vi "Autonomous Independent.vi"   [LabVIEW 2018]
doc: "This VI is called when autonomous begins, and will automatically be terminated when autonomous ends. You can carry out timed or sensor driven robot movement independently without needing to return to the caller."
uses:
  <vilib>/Rock Robotics/WPI/Utilities/WPI_GetSetVariantRefNum.vi
  <vilib>/Rock Robotics/Network Tables/NT Read String.vi
  <vilib>/Rock Robotics/Network Tables/NT Write Numeric Array.vi
panel:
  # "Be sure to right-click and choose Data Operations>>Make Current Value default if you want to save the array values with the VI"
types:
  T1 = typedef "WPI_JoystickDevRef.ctl" = cluster{"Device":T2}
  T2 = typedef "WPI_JoystickDeviceEnum.ctl" = enum16{"USB 0", "USB 1", "USB 2", "USB 3", "USB 4", "USB 5"}
  T3 = cluster{"Gyro":string, "Mtr 1":string, "Mtr 2":string}
  T4 = typedef "WPI_RobotDriveDevRef.ctl" = cluster{"DevStatus":errorcluster, "Motors[]":T5[], "Square Inputs":bool, "Max Output":dbl}
  T5 = typedef "WPI_MotorControlDeviceRef.ctl" = cluster{"DeviceStatus":errorcluster, "Type":T6, "PWM":cluster{"PWM Channel":T7, "DeadBand":T8}, "CAN":cluster{"Device Number":u8, "SetOutput VI Ref":variant, "GetOutput VI Ref":variant, "Enable VI Ref":variant, "Disable VI Ref":variant, "Data":variant}, "Invert":bool, "DIO PWM":cluster{"PWM \"Enable\" Channel":T7, "DIOChannel":T9, "PWM Rate":dbl}}
  T6 = typedef "WPI_MotorControlType.ctl" = enum16{"PWM", "CAN", "DIO PWM"}
  T7 = typedef "FPGA_DIOPWMChannel.ctl" = enum8{"PWM 0", "PWM 1", "PWM 2", "PWM 3", "PWM 4", "PWM 5", "PWM 6", "PWM 7", "PWM 8", "PWM 9", "PWM MXP 0", "PWM MXP 1", "PWM MXP 2", "PWM MXP 3", "PWM MXP 4", "PWM MXP 5", "PWM MXP 6", "PWM MXP 7", "PWM MXP 8", "PWM MXP 9", "Invalid"}
  T8 = typedef "WPI_PWMDeadband.ctl" = cluster{"Name":string, "maxPositivePwm":i32, "minPositivePwm":i32, "centerPwm":i32, "maxNegativePwm":i32, "minNegativePwm":i32, "angularRange":u16}
  T9 = typedef "FPGA_DIOChannel.ctl" = enum8{"DIO 0", "DIO 1", "DIO 2", "DIO 3", "DIO 4", "DIO 5", "DIO 6", "DIO 7", "DIO 8", "DIO 9", "DIO MXP 0", "DIO MXP 1", "DIO MXP 2", "DIO MXP 3", "DIO MXP 4", "DIO MXP 5", "DIO MXP 6", "DIO MXP 7", "DIO MXP 8", "DIO MXP 9", "DIO MXP 10", "DIO MXP 11", "DIO MXP 12", "DIO MXP 13", "DIO MXP 14", "DIO MXP 15", "SPI Port CS1", "SPI Port CS2", "SPI Port CS3", "SPI Port MISO", "SPI Port MOSI", "Invalid"}
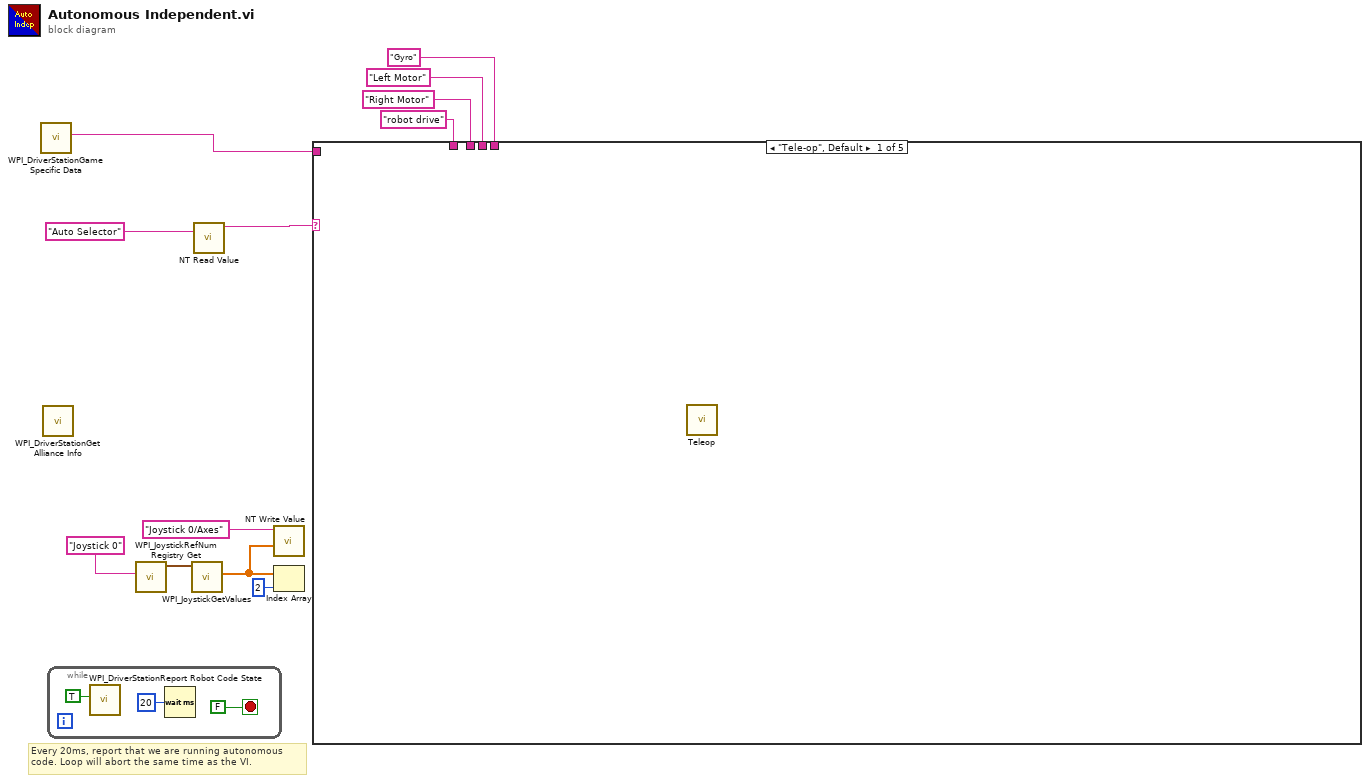
[diagram p0: block diagram]
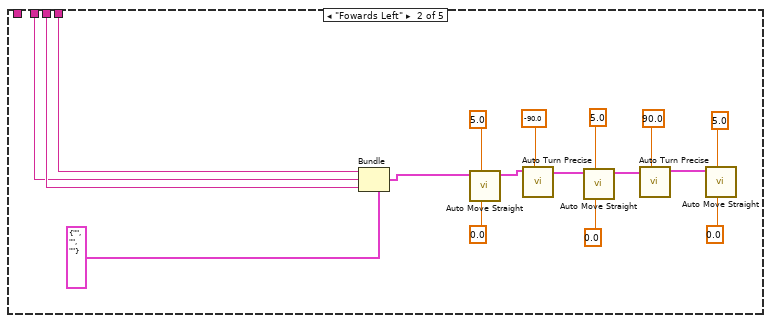
[diagram p2: hidden frame]
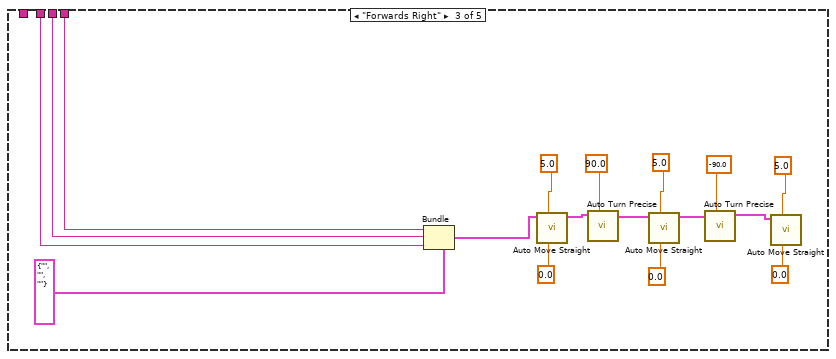
[diagram p3: hidden frame]
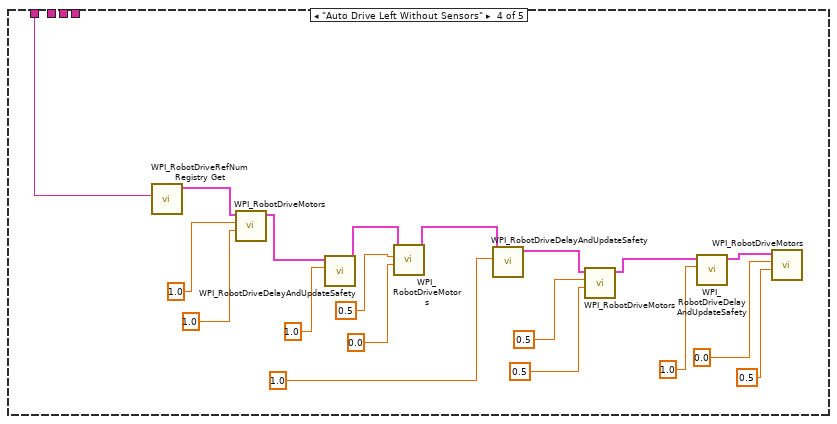
[diagram p4: hidden frame]
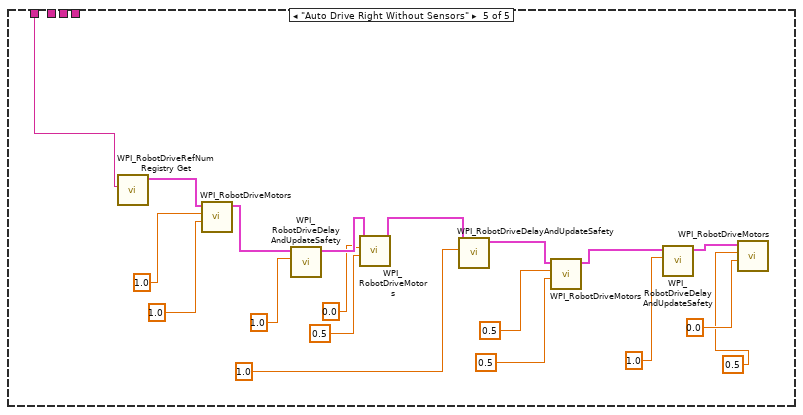
[diagram p5: hidden frame]
diagram:
  # "Every 20ms, report that we are running autonomous\ncode. Loop will abort the same time as the VI."
  n1 = call <vilib>:"WPI_DriverStationGame Specific Data.vi"() -> ("Game Specific Data"=w5:string)  [unwired: 11 in]
  n2 = call <vilib>:"WPI_DriverStationGet Alliance Info.vi"() -> ()  [unwired: 12 out]
  n3 = while {
    stop <- FALSE stop-if-true
    n4 = call <vilib>:"WPI_DriverStationReport Robot Code State.vi"("Autonomous"=TRUE) -> ()  [unwired: 10 in, 1 out]
    n5 = Wait (ms)(milliseconds to wait=u32 20) -> ()  [unwired: 1 out]
  }
  n6 = call <vilib>:"WPI_JoystickRefNum Registry Get.vi"("refnum name"="Joystick 0") -> ("JoystickDevRef"=w11:T1)  [unwired: 1 in, 9 out]
  n7 = call <vilib>:"WPI_JoystickGetValues.vi"("JoystickDevRef"=w11) -> ("Axes"=w7:dbl[])  [unwired: 6 in, 4 out]
  n8 = call-poly <vilib>:"NT Read Value.vi"("Name"="Auto Selector") -> ("String"=w8:string)  [unwired: 9 in, 1 out]
  n9 = call-poly <vilib>:"NT Write Value.vi"("Numeric Array"=w7, "Name"="Joystick 0/Axes") -> ()  [unwired: 9 in, 1 out]
  n10 = Index Array(array=w7, index=2) -> ()  [unwired: 1 out]
  n11 = case shown="\"Tele-op\", Default" w8 {
    tunnel: w5 -> [_ _ _ _ _]
    tunnel: "robot drive" ("refnum name") -> [_ _ _ w50 w69]
    tunnel: "Gyro" ("refnum name") -> [_ w18 w35 _ _]
    tunnel: "Left Motor" ("refnum name") -> [_ w17 w33 _ _]
    tunnel: "Right Motor" ("refnum name") -> [_ w16 w34 _ _]
    frame "Tele-op", Default {
      n12 = call "Teleop.vi"() -> ()  [unwired: 3 in, 9 out]
    }
    frame "Fowards Left" {
      n13 = Bundle(cluster=T3 {"Gyro"="", "Mtr 1"="", "Mtr 2"=""} ("Refnum's In"), "Gyro"=w18, "Mtr 1"=w16, "Mtr 2"=w17) -> (w21:T3)
      n14 = call "Auto Move Straight.vi"("Target Angle"=0.0, "Target Distance"=5.0, "Refnum's In"=w21) -> ("Refnum's Out"=w29:T3)  [unwired: 7 in, 1 out]
      n15 = call "Auto Turn Precise.vi"("Target Distance"=-90.0, "Refnum's In"=w29) -> ("Refnum's Out"=w28:T3)  [unwired: 8 in, 1 out]
      n16 = call "Auto Move Straight.vi"("Target Angle"=0.0, "Target Distance"=5.0, "Refnum's In"=w28) -> ("Refnum's Out"=w26:T3)  [unwired: 7 in, 1 out]
      n17 = call "Auto Turn Precise.vi"("Target Distance"=90.0, "Refnum's In"=w26) -> ("Refnum's Out"=w24:T3)  [unwired: 8 in, 1 out]
      n18 = call "Auto Move Straight.vi"("Target Angle"=0.0, "Target Distance"=5.0, "Refnum's In"=w24) -> ()  [unwired: 7 in, 2 out]
    }
    frame "Forwards Right" {
      n19 = Bundle(cluster=T3 {"Gyro"="", "Mtr 1"="", "Mtr 2"=""} ("Refnum's In"), "Gyro"=w35, "Mtr 1"=w34, "Mtr 2"=w33) -> (w45:T3)
      n20 = call "Auto Move Straight.vi"("Target Angle"=0.0, "Target Distance"=5.0, "Refnum's In"=w45) -> ("Refnum's Out"=w44:T3)  [unwired: 7 in, 1 out]
      n21 = call "Auto Turn Precise.vi"("Target Distance"=90.0, "Refnum's In"=w44) -> ("Refnum's Out"=w43:T3)  [unwired: 8 in, 1 out]
      n22 = call "Auto Move Straight.vi"("Target Angle"=0.0, "Target Distance"=5.0, "Refnum's In"=w43) -> ("Refnum's Out"=w40:T3)  [unwired: 7 in, 1 out]
      n23 = call "Auto Turn Precise.vi"("Target Distance"=-90.0, "Refnum's In"=w40) -> ("Refnum's Out"=w38:T3)  [unwired: 8 in, 1 out]
      n24 = call "Auto Move Straight.vi"("Target Angle"=0.0, "Target Distance"=5.0, "Refnum's In"=w38) -> ()  [unwired: 7 in, 2 out]
    }
    frame "Auto Drive Left Without Sensors" {
      n25 = call <vilib>:"WPI_RobotDriveRefNum Registry Get.vi"("refnum name"=w50) -> ("RobotDriveDevRef"=w61:T4)  [unwired: 9 in, 1 out]
      n26 = call <vilib>:"WPI_RobotDriveMotors.vi"("RightSpeed"=1.0 ("Y axis value"), "LeftSpeed"=1.0 ("X axis value"), "RobotDriveDevRef"=w61) -> ("RobotDriveDevRef"=w60:T4)  [unwired: 6 in, 2 out]
      n27 = call <vilib>:"WPI_RobotDriveDelayAndUpdateSafety.vi"("Delay (s)"=1.0, "RobotDriveDevRef"=w60) -> ("RobotDriveDevRef 2"=w65:T4)  [unwired: 8 in, 1 out]
      n28 = call <vilib>:"WPI_RobotDriveMotors.vi"("RightSpeed"=0.0 ("Y axis value"), "LeftSpeed"=0.5 ("X axis value"), "RobotDriveDevRef"=w65) -> ("RobotDriveDevRef"=w64:T4)  [unwired: 6 in, 2 out]
      n29 = call <vilib>:"WPI_RobotDriveDelayAndUpdateSafety.vi"("Delay (s)"=1.0, "RobotDriveDevRef"=w64) -> ("RobotDriveDevRef 2"=w57:T4)  [unwired: 8 in, 1 out]
      n30 = call <vilib>:"WPI_RobotDriveMotors.vi"("RightSpeed"=0.5 ("Y axis value"), "LeftSpeed"=0.5 ("X axis value"), "RobotDriveDevRef"=w57) -> ("RobotDriveDevRef"=w56:T4)  [unwired: 6 in, 2 out]
      n31 = call <vilib>:"WPI_RobotDriveDelayAndUpdateSafety.vi"("Delay (s)"=1.0, "RobotDriveDevRef"=w56) -> ("RobotDriveDevRef 2"=w51:T4)  [unwired: 8 in, 1 out]
      n32 = call <vilib>:"WPI_RobotDriveMotors.vi"("RightSpeed"=0.5 ("Y axis value"), "LeftSpeed"=0.0 ("X axis value"), "RobotDriveDevRef"=w51) -> ()  [unwired: 6 in, 3 out]
    }
    frame "Auto Drive Right Without Sensors" {
      n33 = call <vilib>:"WPI_RobotDriveRefNum Registry Get.vi"("refnum name"=w69) -> ("RobotDriveDevRef"=w80:T4)  [unwired: 9 in, 1 out]
      n34 = call <vilib>:"WPI_RobotDriveMotors.vi"("RightSpeed"=1.0 ("Y axis value"), "LeftSpeed"=1.0 ("X axis value"), "RobotDriveDevRef"=w80) -> ("RobotDriveDevRef"=w79:T4)  [unwired: 6 in, 2 out]
      n35 = call <vilib>:"WPI_RobotDriveDelayAndUpdateSafety.vi"("Delay (s)"=1.0, "RobotDriveDevRef"=w79) -> ("RobotDriveDevRef 2"=w84:T4)  [unwired: 8 in, 1 out]
      n36 = call <vilib>:"WPI_RobotDriveMotors.vi"("RightSpeed"=0.5 ("Y axis value"), "LeftSpeed"=0.0 ("X axis value"), "RobotDriveDevRef"=w84) -> ("RobotDriveDevRef"=w83:T4)  [unwired: 6 in, 2 out]
      n37 = call <vilib>:"WPI_RobotDriveDelayAndUpdateSafety.vi"("Delay (s)"=1.0, "RobotDriveDevRef"=w83) -> ("RobotDriveDevRef 2"=w76:T4)  [unwired: 8 in, 1 out]
      n38 = call <vilib>:"WPI_RobotDriveMotors.vi"("RightSpeed"=0.5 ("Y axis value"), "LeftSpeed"=0.5 ("X axis value"), "RobotDriveDevRef"=w76) -> ("RobotDriveDevRef"=w75:T4)  [unwired: 6 in, 2 out]
      n39 = call <vilib>:"WPI_RobotDriveDelayAndUpdateSafety.vi"("Delay (s)"=1.0, "RobotDriveDevRef"=w75) -> ("RobotDriveDevRef 2"=w70:T4)  [unwired: 8 in, 1 out]
      n40 = call <vilib>:"WPI_RobotDriveMotors.vi"("RightSpeed"=0.0 ("Y axis value"), "LeftSpeed"=0.5 ("X axis value"), "RobotDriveDevRef"=w70) -> ()  [unwired: 6 in, 3 out]
    }
  }
